vi "is visible to load.vi"(8 "error in":errorcluster, 11 "Shared Library Module editor node in":refnum<class "Shared Library Module editor node.lvclass">) -> (0 "error out":errorcluster, 2 "visible":bool, 3 "Shared Library Module editor node out":refnum<class "Shared Library Module editor node.lvclass">)   [LabVIEW 2013, in "Shared Library Module editor node.lvclass"]
doc: "Determines whether a node should be visible when generating right click menus. By default, any abstract node is not visible."
uses:
  Shared Library Module editor node.lvclass
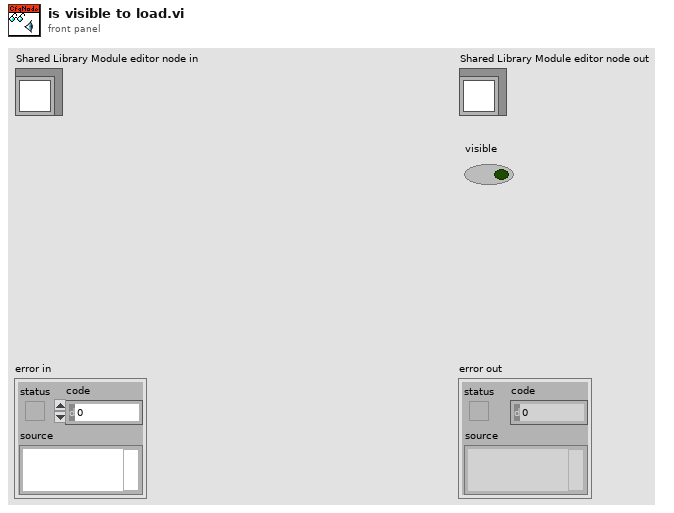
[diagram p1: front panel]
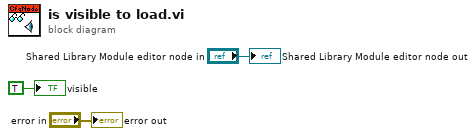
[diagram p0: block diagram]
diagram:
  "error out" <- "error in"
  "Shared Library Module editor node out" <- "Shared Library Module editor node in"
  "visible" <- TRUE ("visible")
